vi "Read Error Handler Interface.vi"(8 "error in (no error)":errorcluster, 11 "Error Handler Interface Test in":refnum<class "Error Handler Interface Test.lvclass">) -> (0 "error out":errorcluster, 2 "Error Handler Interface":refnum<class "Error Handler Interface.lvclass">, 3 "Error Handler Interface Test out":refnum<class "Error Handler Interface Test.lvclass">)   [LabVIEW 2020, in "Error Handler Interface Test.lvclass"]
uses:
  Error Handler Interface Test.lvclass
  Framework/Error Handler Interface/Error Handler Interface.lvclass
  Error Handler Interface Test.lvclass/Error Handler Interface Test.ctl
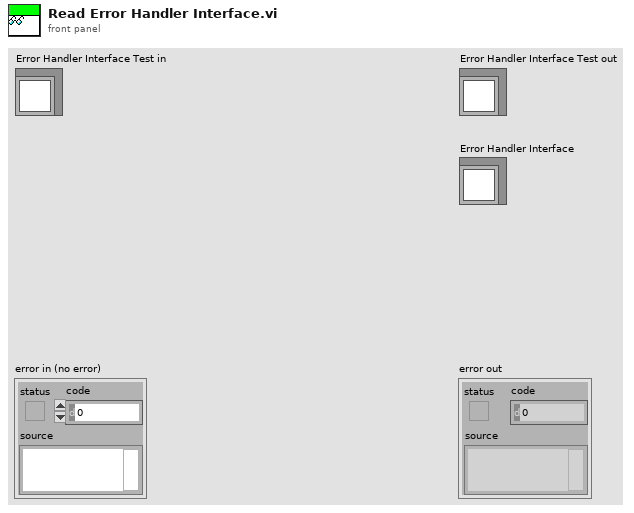
[diagram p1: front panel]
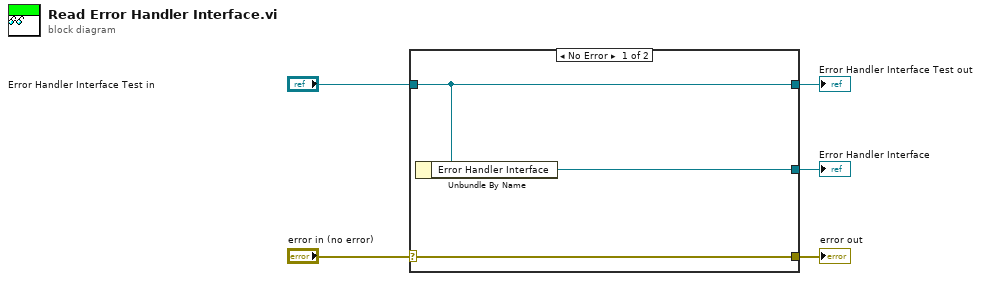
[diagram p0: block diagram]
diagram:
  n1 = case shown="No Error" "error in (no error)" {
    selector: "error in (no error)" -> [w8 w9]
    tunnel: [w8 w9] -> w4
    tunnel: [w7 w10] -> w2
    tunnel: "Error Handler Interface Test in" -> [w7 w10]
    tunnel: [w6 _] -> w1
    frame No Error {
      n2 = Unbundle By Name(w7) -> ("Error Handler Interface"=w6:refnum<class "Error Handler Interface.lvclass">)
    }
    frame Error {
    }
  }
  "error out" <- w4
  "Error Handler Interface Test out" <- w2
  "Error Handler Interface" <- w1
